vi "RW_Mutex_Give.vi"(10 "error in (no error)":errorcluster) -> (2 "error out":errorcluster)   [LabVIEW 2016]
uses:
  RW_Mutex.vi
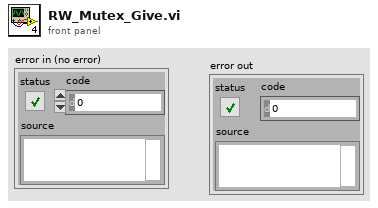
[diagram p1: front panel]
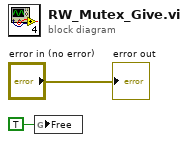
[diagram p0: block diagram]
diagram:
  n1 = global write "RW_Mutex.vi" "Free"(TRUE ("Free")) -> ()
  "error out" <- "error in (no error)"
